vi "Get package_templatemessage.vi"(8 "error in (no error)":errorcluster, 11 "gRPCid":T1) -> (0 "error out":errorcluster, 2 "package_templatemessage":T2, 3 "gRPCid out":T1)   [LabVIEW 2024, in "Service Template.lvlib"]
uses:
  Service Template.lvlib
  package_templatemessage.ctl
  c750bf2f-d32b-4a25-a00a-5db67bc240fd.vi
  2ed25e12-861d-4677-8ead-ace2906b2041.vi
  gRPC lv Support/grpc-lvsupport/grpcId.ctl
  gRPC lv Support/grpc-lvsupport/grpc-lvsupport.lvlib
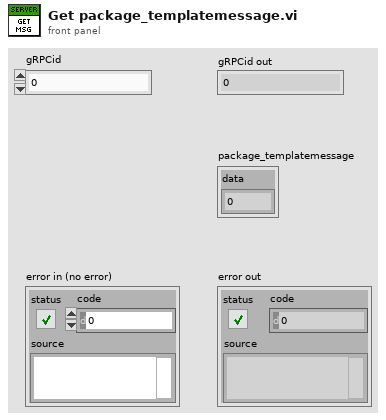
[diagram p1: front panel]
types:
  T1 = typedef "grpc-lvsupport.lvlib/grpcId.ctl" = u64
  T2 = typedef "Service Template.lvlib/package_templatemessage.ctl" = cluster{"data":sgl}
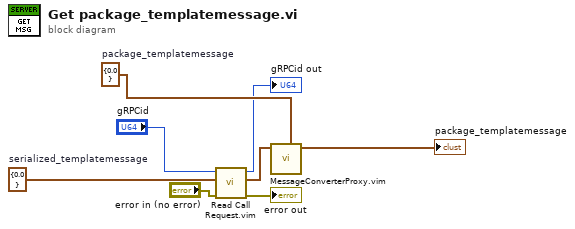
[diagram p0: block diagram]
diagram:
  w6 = T2 {"data"=0.0}  # serialized_templatemessage
  w5 = T2 {"data"=0.0}  # package_templatemessage
  n1 = call "Read Call Request.vim"("error in"="error in (no error)", "Request Type"=w6, "gRPCid in"="gRPCid") -> ("error out"=→"error out":errorcluster, "Request Data"=w4:T2, "gRPCid out"=→"gRPCid out":T1)  [unwired: 6 in]
  n2 = call "MessageConverterProxy.vim"("package_templatemessage_type"=w5, "example_SignalParameters_Data"=w4) -> ("package_templatemessage"=→"package_templatemessage":T2)  [unwired: 9 in]
